vi "Edit Chassis_Edit Chassis.vi"(8 "error in (no error)":errorcluster, 10 "Settings":T1={"Name"="", "Master Chassis"={"Type"=enum."None", "DAQ Name"="", "clkSrc"=10280, "activeEdge"=0, "exportClk"=0, "exportClkToLine"=0, "triggerLine"=10171, "triggerSlope"=0, "startTrigger"=0, "startTriggerLine"=0}} {"Master Chassis"."startTriggerLine" items=["None", "PFI_0", "PFI_1", "PFI_2", "PFI_3", "PFI_4", "PFI_5", "PFI_6", "PFI_7", "PFI_8", "PFI_9", "PFI_10", "PFI_11", "PFI_12", "PFI_13", "PFI_14", "PFI_15", "RTSI_PXI_TRIG_0", "RTSI_PXI_TRIG_1", "RTSI_PXI_TRIG_2", "RTSI_PXI_TRIG_3", "RTSI_PXI_TRIG_4", "RTSI_PXI_TRIG_5", "RTSI_PXI_TRIG_6", "RTSI_PXI_TRIG_7"]; "Master Chassis"."startTrigger" items=["aiStartTrigger", "aoStartTrigger"]; "Master Chassis"."triggerSlope" items=["Falling"=10171, "Rising"=10280]; "Master Chassis"."triggerLine" items=["None", "PFI_0", "PFI_1", "PFI_2", "PFI_3", "PFI_4", "PFI_5", "PFI_6", "PFI_7", "PFI_8", "PFI_9", "PFI_10", "PFI_11", "PFI_12", "PFI_13", "PFI_14", "PFI_15", "RTSI_PXI_TRIG_0", "RTSI_PXI_TRIG_1", "RTSI_PXI_TRIG_2", "RTSI_PXI_TRIG_3", "RTSI_PXI_TRIG_4", "RTSI_PXI_TRIG_5", "RTSI_PXI_TRIG_6", "RTSI_PXI_TRIG_7"]; "Master Chassis"."exportClkToLine" items=["Default_RTSI_PXI_TRIG_0", "PFI_0", "PFI_1", "PFI_2", "PFI_3", "PFI_4", "PFI_5", "PFI_6", "PFI_7", "PFI_8", "PFI_9", "PFI_10", "PFI_11", "PFI_12", "PFI_13", "PFI_14", "PFI_15", "RTSI_PXI_TRIG_0", "RTSI_PXI_TRIG_1", "RTSI_PXI_TRIG_2", "RTSI_PXI_TRIG_3", "RTSI_PXI_TRIG_4", "RTSI_PXI_TRIG_5", "RTSI_PXI_TRIG_6", "RTSI_PXI_TRIG_7"]; "Master Chassis"."exportClk" items=["aiSampleClock", "aoSampleClock"]; "Master Chassis"."activeEdge" items=["Falling"=10171, "Rising"=10280]; "Master Chassis"."clkSrc" items=["Onboard10MHzClock", "PFI_0", "PFI_1", "PFI_2", "PFI_3", "PFI_4", "PFI_5", "PFI_6", "PFI_7", "PFI_8", "PFI_9", "PFI_10", "PFI_11", "PFI_12", "PFI_13", "PFI_14", "PFI_15", "RTSI_PXI_TRIG_0", "RTSI_PXI_TRIG_1", "RTSI_PXI_TRIG_2", "RTSI_PXI_TRIG_3", "RTSI_PXI_TRIG_4", "RTSI_PXI_TRIG_5", "RTSI_PXI_TRIG_6", "RTSI_PXI_TRIG_7"]}, 11 "Chassis Ref":refnum<k24>) -> (0 "error out":errorcluster, 3 "Chassis Ref Out":refnum<k24>)   [LabVIEW 2019, in "Simple SysDef API.lvlib"]
uses:
  <userlib>/SimpleSysDef/Simple SysDef API.lvlib
  NationalInstruments.VeriStand.SystemDefinitionAPI
  <userlib>/SimpleSysDef/_SubVIs/Edit Chassis_Settings.ctl
  <userlib>/SimpleSysDef/_SubVIs/Add Chassis_DAQ Master Settings.ctl
  <userlib>/SimpleSysDef/_SubVIs/Add Chassis_Type.ctl
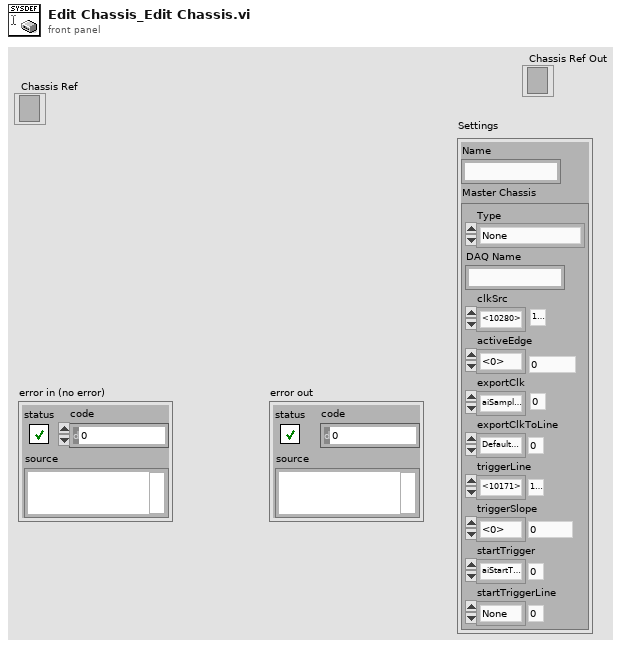
[diagram p1: front panel]
types:
  T1 = typedef "Simple SysDef API.lvlib/Edit Chassis_Settings.ctl" = cluster{"Name":string, "Master Chassis":T2}
  T2 = typedef "Simple SysDef API.lvlib/Add Chassis_DAQ Master Settings.ctl" = cluster{"Type":T3, "DAQ Name":string, "clkSrc":i32, "activeEdge":i32, "exportClk":i32, "exportClkToLine":i32, "triggerLine":i32, "triggerSlope":i32, "startTrigger":i32, "startTriggerLine":i32}
  T3 = typedef "Simple SysDef API.lvlib/Add Chassis_Type.ctl" = enum16{"None", "DAQ", "FPGA", "Timing and Sync", "Automatic"}
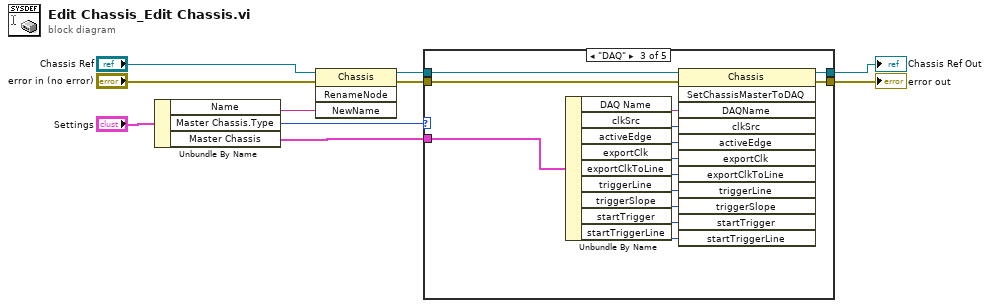
[diagram p0: block diagram]
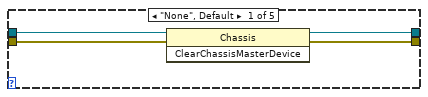
[diagram p2: hidden frame]
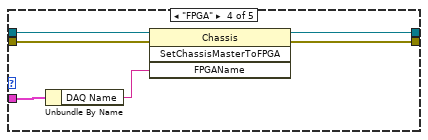
[diagram p4: hidden frame]
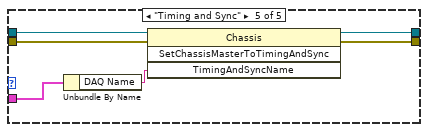
[diagram p5: hidden frame]
diagram:
  n1 = Unbundle By Name("Settings") -> ("Name"=w5:string, "Master Chassis.Type"=w9:T3, "Master Chassis"=w8:T2)
  n2 = invoke class="Chassis" method="RenameNode"(reference="Chassis Ref", error in="error in (no error)", "NewName"=w5) -> (reference out=w2:refnum<k24>, error out=w6:errorcluster)  [unwired: 1 in, 2 out]
  n3 = case shown="\"DAQ\"" w9 {
    tunnel: w2 -> [w14 w16 w30 w36 w42]
    tunnel: w6 -> [w12 w15 w17 w31 w37]
    tunnel: [w13 w16 w29 w35 w41] -> w3
    tunnel: [w11 w15 w28 w34 w40] -> w4
    tunnel: w8 -> [_ _ w18 w33 w39]
    frame "None", Default {
      n4 = invoke class="Chassis" method="ClearChassisMasterDevice"(reference=w14, error in=w12) -> (reference out=w13:refnum<k24>, error out=w11:errorcluster)  [unwired: 1 in, 1 out]
    }
    frame "Automatic" {
    }
    frame "DAQ" {
      n5 = Unbundle By Name(w18) -> ("DAQ Name"=w27:string, "clkSrc"=w26:i32, "activeEdge"=w25:i32, "exportClk"=w24:i32, "exportClkToLine"=w23:i32, "triggerLine"=w22:i32, "triggerSlope"=w21:i32, "startTrigger"=w20:i32, "startTriggerLine"=w19:i32)
      n6 = invoke class="Chassis" method="SetChassisMasterToDAQ"(reference=w30, error in=w17, "DAQName"=w27, "clkSrc"=w26, "activeEdge"=w25, "exportClk"=w24, "exportClkToLine"=w23, "triggerLine"=w22, "triggerSlope"=w21, "startTrigger"=w20, "startTriggerLine"=w19) -> (reference out=w29:refnum<k24>, error out=w28:errorcluster)  [unwired: 1 in, 10 out]
    }
    frame "FPGA" {
      n7 = Unbundle By Name(w33) -> ("DAQ Name"=w32:string)
      n8 = invoke class="Chassis" method="SetChassisMasterToFPGA"(reference=w36, error in=w31, "FPGAName"=w32) -> (reference out=w35:refnum<k24>, error out=w34:errorcluster)  [unwired: 1 in, 2 out]
    }
    frame "Timing and Sync" {
      n9 = Unbundle By Name(w39) -> ("DAQ Name"=w38:string)
      n10 = invoke class="Chassis" method="SetChassisMasterToTimingAndSync"(reference=w42, error in=w37, "TimingAndSyncName"=w38) -> (reference out=w41:refnum<k24>, error out=w40:errorcluster)  [unwired: 1 in, 2 out]
    }
  }
  "error out" <- w4
  "Chassis Ref Out" <- w3
